vi "safe digital outputs.vi"(9 "Message handler data":T1) -> (0 "error out":errorcluster)   [LabVIEW 2018]
uses:
  Type Defs/Message loop data.ctl
  Type Defs/FPGA reference.ctl
  Type Defs/RT Status.ctl
  <vilib>/Utility/error.llb/Error Cluster From Error Code.vi
  <vilib>/rvi/errors/niLvFpgaAdjustHostInterfaceError.vi
  <vilib>/rvi/interface/nirviReadWriteControl/nirviReadWriteControl.xnode
  FPGA Bitfiles/CompressorRigV2_CompressorFPGA_FPGAMainV3_7sPRekuravM.lvbitx
  NiFpgaLv.dll
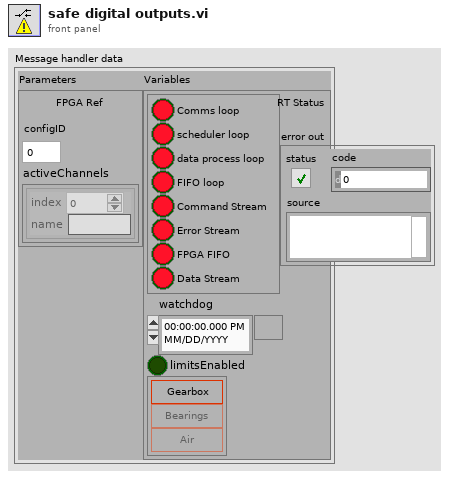
[diagram p1: front panel]
types:
  T1 = typedef "Message loop data.ctl" = cluster{"Parameters":cluster{"FPGA Ref":T2, "configID":u32, "activeChannels":cluster{"index":u16, "name":string}[]}, "Variables":cluster{"RT Status":T3, "watchdog":timestamp, "limitsEnabled":bool, "Interlocks":cluster{"gearboxOil":bool, "bearingOil":bool, "gearboxAir":bool}}}
  T2 = typedef "FPGA reference.ctl" = refnum<k20>
  T3 = typedef "RT Status.ctl" = cluster{"Comms loop":bool, "scheduler loop":bool, "data process loop":bool, "FIFO loop":bool, "Command Stream":bool, "Error Stream":bool, "FPGA FIFO":bool, "Data Stream":bool}
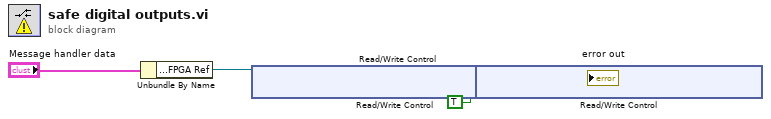
[diagram p0: block diagram]
diagram:
  n1 = Unbundle By Name("Message handler data") -> ("Parameters.FPGA Ref"=w8:T2)
  n2 = xnode "Read/Write Control"("FPGA VI Reference In"=w8) -> ("FPGA VI Reference Out"=w5:T2, "error out"=w3:errorcluster, "Safe Digital"=w4:bool[])  [unwired: 1 in]
  n3 = xnode "Read/Write Control"("FPGA VI Reference In"=w5, "error in"=w3, "Safe Digital"=w4) -> ("FPGA VI Reference Out"=w7:T2, "error out"=w2:errorcluster)
  n4 = xnode "Read/Write Control"("FPGA VI Reference In"=w7, "error in"=w2, "Update Outputs"=TRUE ("Enable Data FIFO")) -> ("error out"=→"error out":errorcluster)  [unwired: 1 out]
